vi "Database New.vi"(8 "error in (no error)":errorcluster, 10 "Database File Path":path, 11 "object in":refnum<class "Database.lvclass">) -> (0 "error out":errorcluster, 3 "object out":refnum<class "Database.lvclass">)   [LabVIEW 2015, in "Database.lvclass"]
uses:
  Database.lvclass
  Database.lvclass/Database.ctl
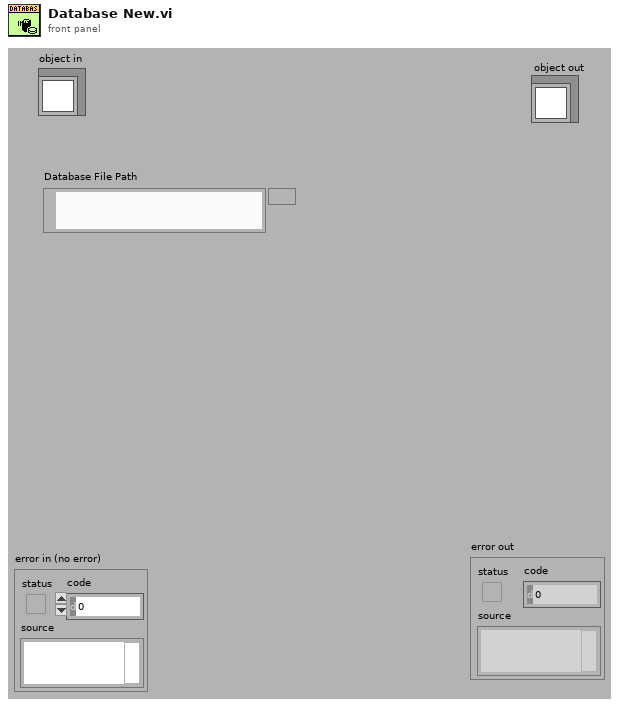
[diagram p1: front panel]
types:
  T1 = enum16{"open", "replace", "create", "open or create", "replace or create", "replace or create with confirmation"}
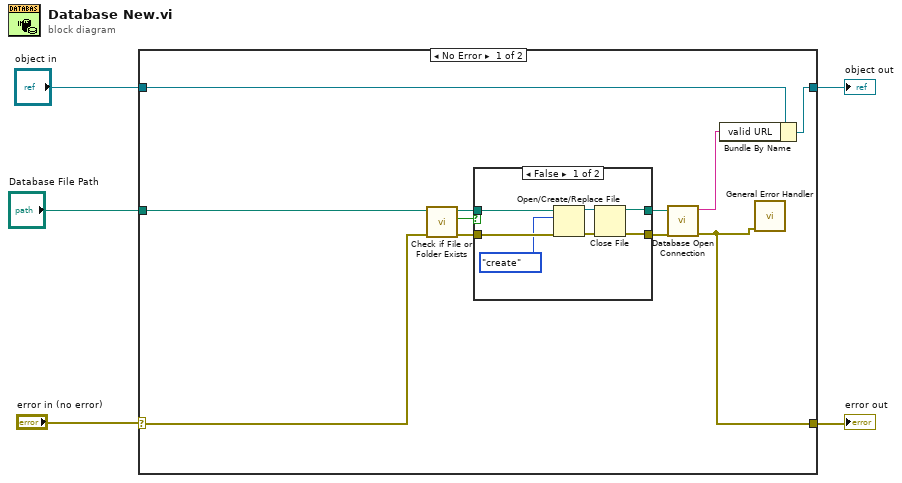
[diagram p0: block diagram]
diagram:
  n1 = case shown="No Error" "error in (no error)" {
    selector: "error in (no error)" -> [w16 w26]
    tunnel: "object in" -> [w11 w27]
    tunnel: [w9 w27] -> w4
    tunnel: [w8 w26] -> w2
    tunnel: "Database File Path" -> [w6 _]
    frame No Error {
      n2 = call <vilib>:"Check if File or Folder Exists.vi"("error in (no error)"=w16, "path"=w6) -> ("error out"=w13:errorcluster, "file or folder exists?"=w15:bool, "dup path"=w14:path)  [unwired: 7 in]
      n3 = case shown="False" w15 {
        tunnel: w14 -> [w23 w25]
        tunnel: w13 -> [w22 w24]
        tunnel: [w18 w25] -> w7
        tunnel: [w17 w24] -> w12
        frame False {
          n4 = Open/Create/Replace File(file path (use dialog)=w23, error in=w22, operation (0:open)=T1."create") -> (refnum out=w20:refnum<file>, error out=w19:errorcluster)  [unwired: 3 in, 1 out]
          n5 = Close File(refnum=w20, error in=w19) -> (path=w18:path, error out=w17:errorcluster)
        }
        frame True {
          # "It has exit!"
        }
      }
      n6 = call "Database Open Connection.vi"("error in"=w12, "Database File Path"=w7) -> ("error out"=w8:errorcluster, "valid URL"=w10:string)  [unwired: 8 in]
      n7 = Bundle By Name(cluster=w11, "valid URL"=w10) -> (w9:refnum<class "Database.lvclass">)
      n8 = call <vilib>:"General Error Handler.vi"("error in (no error)"=w8) -> ()  [unwired: 10 in, 5 out]
    }
    frame Error {
    }
  }
  "object out" <- w4
  "error out" <- w2
